vi "Init.vi"(8 "error in (no error)":errorcluster, 9 "GRR Result Session":string, 10 "STDF Parser":string, 11 "GRR Core in":refnum<class "GRR Core.lvclass">) -> (0 "error out":errorcluster, 3 "GRR Core out":refnum<class "GRR Core.lvclass">)   [LabVIEW 2018, in "GRR Core.lvclass"]
uses:
  GRR Core.lvclass
  GRR Core.lvclass/GRR Core.ctl
  TestDataMgr/TestDataMgr.lvclass
  Result Data Mgr/Result Data Mgr.lvclass
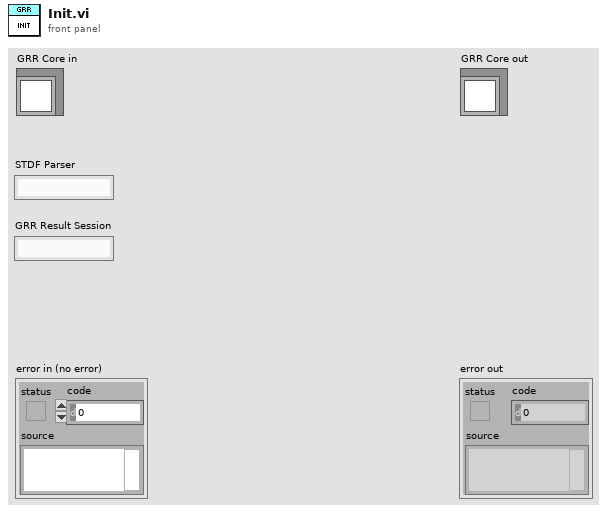
[diagram p1: front panel]
types:
  T1 = typedef "TestDataMgr.lvclass/Session Handle.ctl" = refnum<data-value>
  T2 = typedef "Result Data Mgr.lvclass/Session Handle.ctl" = refnum<data-value>
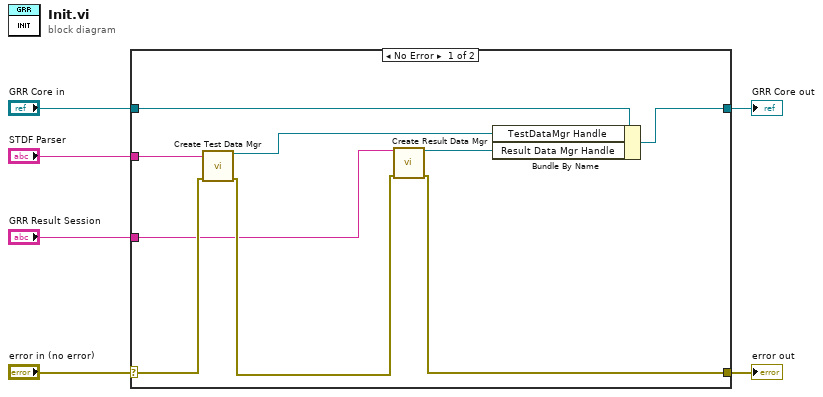
[diagram p0: block diagram]
diagram:
  n1 = case shown="No Error" "error in (no error)" {
    selector: "error in (no error)" -> [w14 w17]
    tunnel: [w7 w17] -> w5
    tunnel: [w8 w16] -> w3
    tunnel: "GRR Core in" -> [w11 w16]
    tunnel: "STDF Parser" -> [w15 _]
    tunnel: "GRR Result Session" -> [w12 _]
    frame No Error {
      n2 = call "Create Test Data Mgr.vi"("Session  Name ()"=w15, "error in (no error)"=w14) -> ("Session Handle"=w10:T1, "error out"=w13:errorcluster)  [unwired: 12 in]
      n3 = call "Create Result Data Mgr.vi"("Session  Name ()"=w12, "error in (no error)"=w13) -> ("Session Handle"=w9:T2, "error out"=w7:errorcluster)  [unwired: 12 in]
      n4 = Bundle By Name(cluster=w11, "TestDataMgr Handle"=w10, "Result Data Mgr Handle"=w9) -> (w8:refnum<class "GRR Core.lvclass">)
    }
    frame Error {
    }
  }
  "error out" <- w5
  "GRR Core out" <- w3
